vi "Yokogawa GS200 V output.vi"(2 "VISA resource name":refnum<visa-resource-name>, 3 "Voltage Range (.30 V)":dbl=30.0 min=0.01 max=30.0 format="%.0p", 4 "Enable Auto Range (T: Enable)":bool=TRUE, 5 "Voltage Level (0.0 V)":dbl min=-32.0 max=32.0 format="%.5p", 6 "Enable Output (T: Enable)":bool=TRUE) -> (0 "error out":errorcluster, 1 "VISA resource name out":refnum<visa-resource-name>)   [LabVIEW 2020]
panel:
  in  "error in (no error)":errorcluster
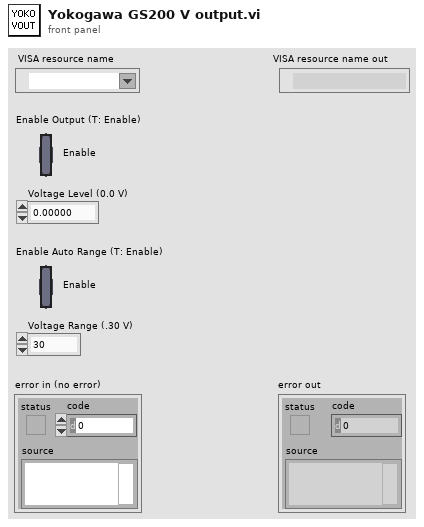
[diagram p1: front panel]
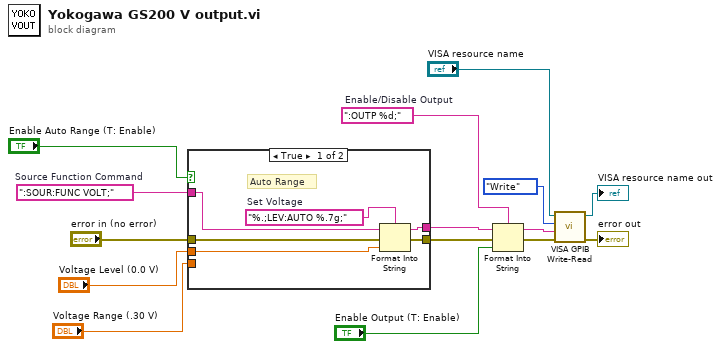
[diagram p0: block diagram]
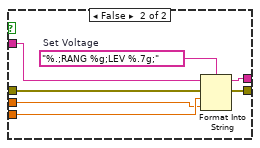
[diagram p2: hidden frame]
diagram:
  w13 = ":OUTP %d;"  # Enable/Disable Output
  w11 = ":SOUR:FUNC VOLT;"  # Source Function Command
  n1 = case shown="True" "Enable Auto Range (T: Enable)" {
    tunnel: "Voltage Level (0.0 V)" -> [w21 w24]
    tunnel: [w19 w27] -> w12
    tunnel: w11 -> [w18 w26]
    tunnel: "Voltage Range (.30 V)" -> [_ w25]
    tunnel: "error in (no error)" -> [w17 w23]
    tunnel: [w16 w22] -> w7
    frame True {
      w20 = "%.;LEV:AUTO %.7g;"  # Set Voltage
      # "Auto Range"
      n2 = Format Into String(format string=w20, initial string=w18, error in=w17, w21) -> (resulting string=w19:string, error out=w16:errorcluster)
    }
    frame False {
      w28 = "%.;RANG %g;LEV %.7g;"  # Set Voltage
      n3 = Format Into String(format string=w28, initial string=w26, error in=w23, w25, w24) -> (resulting string=w27:string, error out=w22:errorcluster)
    }
  }
  n4 = Format Into String(format string=w13, initial string=w12, error in=w7, "Enable Output (T: Enable)") -> (resulting string=w3:string, error out=w2:errorcluster)
  n5 = call "VISA GPIB Write-Read.vi"("error in (no error)"=w2, "Command"=w3, "Action"=enum16{"Write", "Read", "Write & Read"}."Write", "VISA resource name"="VISA resource name") -> ("error out"=→"error out":errorcluster, "dup VISA Session"=→"VISA resource name out":refnum<visa-resource-name>)  [unwired: 4 in, 2 out]
